vi "EtherCAT EnumMasters.vi"(8 "error in (no error)":errorcluster) -> (0 "error out":errorcluster, 1 "masterHdls":T1[](array[typedef]))   [LabVIEW 2017, in "NI_Robotics_KUKA youBot Host.lvlib"]
uses:
  <vilib>/robotics/KUKA youBot/NI_Robotics_KUKA youBot Host.lvlib
  <vilib>/robotics/KUKA youBot/EtherCAT/LowLevel/Mater Handler.ctl
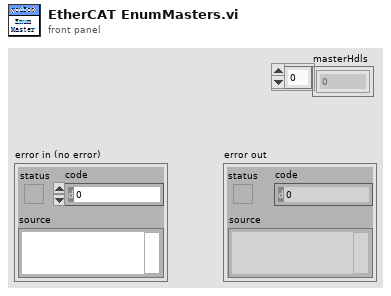
[diagram p1: front panel]
types:
  T1 = typedef "NI_Robotics_KUKA youBot Host.lvlib/Mater Handler.ctl" = i32
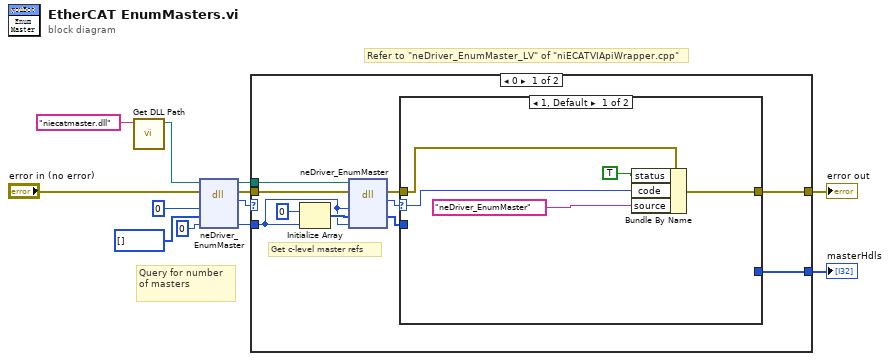
[diagram p0: block diagram]
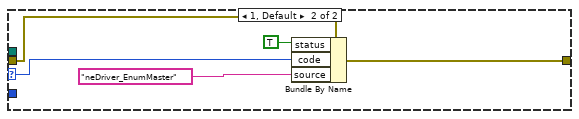
[diagram p3: hidden frame]
diagram:
  # "Refer to \"neDriver_EnumMaster_LV\" of \"niECATVIApiWrapper.cpp\""
  # "Query for number of masters"
  n1 = call <vilib>:"Get DLL Path.vi"("dll name"="niecatmaster.dll") -> ("Path"=w2:path)  [unwired: 10 in]
  n2 = dll-call lib="C:/Program Files (x86)/National Instruments/LabVIEW 2012/resource/Framework/Providers/niecatmaster.dll" fn="neDriver_EnumMaster" ("niecatsv.dll:_neEnumSlaves@16")(path in=w2, error in="error in (no error)", "count"=u32 0, "masterHdls"=i32[] [], "numFetched"=u32 0) -> (path out=w1:path, error out=w5:errorcluster, "return code"=w8:i32, "numFetched"=w7:u32)  [unwired: 1 in, 2 out]
  n3 = case shown="0" w8 {
    selector: w8 -> [_ w32]
    tunnel: w7 -> [w20 _]
    tunnel: [w16 _] -> w6
    tunnel: [w14 w31] -> w4
    tunnel: w5 -> [w15 w30]
    tunnel: w1 -> [w13 _]
    frame 0 {
      # "Get c-level master refs"
      n4 = Initialize Array(0 ("element"), w20) -> (w21:i32[])
      n5 = dll-call lib="C:/Program Files (x86)/National Instruments/LabVIEW 2012/resource/Framework/Providers/niecatmaster.dll" fn="neDriver_EnumMaster" ("niecatsv.dll:_neEnumSlaves@16")(path in=w13, error in=w15, "count"=w20, "masterHdls"=w21, "numFetched"=w20) -> (error out=w19:errorcluster, "return code"=w18:i32, "masterHdls"=w17:i32[])  [unwired: 1 in, 3 out]
      n6 = case shown="1, Default" w18 {
        selector: w18 -> [w25 _]
        tunnel: w19 -> [w23 w28]
        tunnel: w17 -> [_ w29]
        tunnel: [_ w29] -> w16
        tunnel: [w24 w28] -> w14
        frame 1, Default {
          n7 = Bundle By Name(cluster=w23, "status"=TRUE, "code"=w25, "source"="neDriver_EnumMaster") -> (w24:errorcluster)
        }
        frame 0 {
        }
      }
    }
    frame 1, Default {
      n8 = Bundle By Name(cluster=w30, "status"=TRUE, "code"=w32, "source"="neDriver_EnumMaster") -> (w31:errorcluster)
    }
  }
  "error out" <- w4
  "masterHdls" <- w6
